vi "R45_2-FPGA.vi"() -> ()   [LabVIEW 2016]
uses:
  <vilib>/LabVIEW Targets/FPGA/cRIO/shared/nicrio_ModuleControls/nicrio_cRIO-9871_BaudRateEnum.ctl
  <vilib>/LabVIEW Targets/FPGA/cRIO/shared/nicrio_ModuleControls/nicrio_cRIO-9871_DataBitsEnum.ctl
  <vilib>/LabVIEW Targets/FPGA/cRIO/shared/nicrio_ModuleControls/nicrio_cRIO-9871_ParityEnum.ctl
  <vilib>/LabVIEW Targets/FPGA/cRIO/shared/nicrio_ModuleControls/nicrio_cRIO-9871_StopBitsEnum.ctl
  <vilib>/Platform/TimedLoop/XDataNode/timing_clust.ctl
  <vilib>/Platform/TimedLoop/XDataNode/nitl_modes.ctl
  <vilib>/Platform/TimedLoop/XDataNode/wakeup.ctl
  <vilib>/rvi/FXPMathLib/basic elements/FxpIntAccumulator/subVIs/nifxpmath_IntAccumulator_SimConfig.ctl
  <vilib>/rvi/Emulation/niFpgaGetClockAttributes.vi
  <vilib>/rvi/Emulation/niFpgaSctlEmulationGetInTimedLoop.vi
  <vilib>/rvi/Emulation/niFpgaEmulationReportErrorSimple.vi
  <vilib>/rvi/eio/common/nirviEmuTemplateMethod_errors.vi
  <vilib>/rvi/Emulation/niFpgaCriticalErrorInLSC.vi
  <vilib>/rvi/Analysis/common/codeGenErrors/XNode/niFpgaXNodeCodeGenErrorHandle.vi
  <vilib>/rvi/FXPMathLib/basic elements/FxpIntAccumulator/simVIs/DllFxpIntAccumulator_sub.vi
  <vilib>/rvi/eio/common/nirviEmuTemplatePropertySet_errors.vi
  <vilib>/eio/EIONode/EIONode.xnode
  <vilib>/rvi/Analysis/measure/dc-rms/XNode/niFpgaDC-RMS.xnode
  <vilib>/Platform/TimedLoop/XDataNode/XDataNode.xnode
  <vilib>/rvi/FXPMathLib/basic elements/FxpIntAccumulator/XNode/nifxpmath_IntAccumulator.xnode
  <vilib>/rvi/FXPMathLib/FxpMul/XNode/nifxpmath_Multiplier.xnode
  <vilib>/eio/EIOPropertyNode/EIOPropertyNode.xnode
  <vilib>/eio/EIOMethodNode/EIOMethodNode.xnode
  <vilib>/Platform/TimedLoop/XDataNode/XDNodeRunTimeDep.lvlib
  <vilib>/rvi/FXPMathLib/sim/FxpSim.dll
  <vilib>/rvi/eio/common/nirviEmuTemplatePropertyGet_errors.vi
  <vilib>/rvi/eio/common/nirviEmuTemplatePropertyGet_noerrors.vi
  <vilib>/rvi/eio/common/nirviEmuTemplatePropertySet_noerrors.vi
panel:
  out "Vac Cluster 2 interlock error":errorcluster
  out "ExB 2 PS error":errorcluster
  out "Position-Status Sensor error":errorcluster
  out "9485 error":errorcluster
  in  "RT error":bool
  out "R45 Vac Cluster 4 Ion Gauge 2":u8[](array[numeric])
  out "R45 Vac Cluster 4 Convectron 2":u8[](array[numeric])
  out "R45 Vac Cluster 4 Convectron 1":u8[](array[numeric])
  out "R45 Vac Cluster 4 Ion Gauge 1":u8[](array[numeric])
  out "R45 Vacuum Gauge 4 error":errorcluster
  out "R45 Vac Cluster 3 Ion Gauge 2":u8[](array[numeric])
  out "R45 Vac Cluster 3 Convectron 2":u8[](array[numeric])
  out "R45 Vac Cluster 3 Convectron 1":u8[](array[numeric])
  out "R45 Vac Cluster 3 Ion Gauge 1":u8[](array[numeric])
  out "R45 Vacuum Gauge 3 error":errorcluster
  out "R45 Vacuum Gauge 2 error":errorcluster
  out "GFM Hall Probe error":errorcluster
  out "GF ps error":errorcluster
  out "ExB 1 PS error":errorcluster
  out "9264 Error":errorcluster
  out "9205 error":errorcluster
  out "Vac cluster 2 Ion Guage Interlock":bool
  out "Vac cluster 2 Convectron Interlock":bool
  in  "turbo valve R45 ExB":bool
  in  "beamline valve R45 detector":bool
  in  "turbo valve r45 det turbo":bool
  in  "turbo valve r45 waist":bool
  out "Data":u8
  out "Timed Out":bool
  out "GFM read":u8[](array[numeric])
  in  "GFM ps set":u8[](array[numeric])=[0, 0, 0, 0, 0, 0, 0, 0, 0, 0]
  in  "ExB 2 Reset":bool
  in  "ExB 2 PS set":u8[](array[numeric])=[0, 0, 0, 0, 0, 0, 0, 0, 0, 0]
  out "R45 Vac Cluster 2 Ion Gauge 2":u8[](array[numeric])
  out "R45 Vac Cluster 2 Convectron 2":u8[](array[numeric])
  out "R45 Vac Cluster 2 Convectron 1":u8[](array[numeric])
  out "R45 Vac Cluster 2 Ion Gauge 1":u8[](array[numeric])
  in  "ExB 1 PS set":u8[](array[numeric])=[0, 0, 0, 0, 0, 0, 0, 0, 0, 0]
  out "DIO OUTPUT":bool[](array[boolean])
  in  "R45 detector FC insert":bool
  in  "R45 detector Aperture insert":bool
  out "Analog input":fxp<+/-,26,5>[](array[numeric]) format="%.23g"
  in  "Analog Output":fxp<+/-,26,5>[](array[numeric])=[0.0, 0.0, 0.0, 0.0, 0.0, 0.0, 0.0, 0.0] format="%.23g"
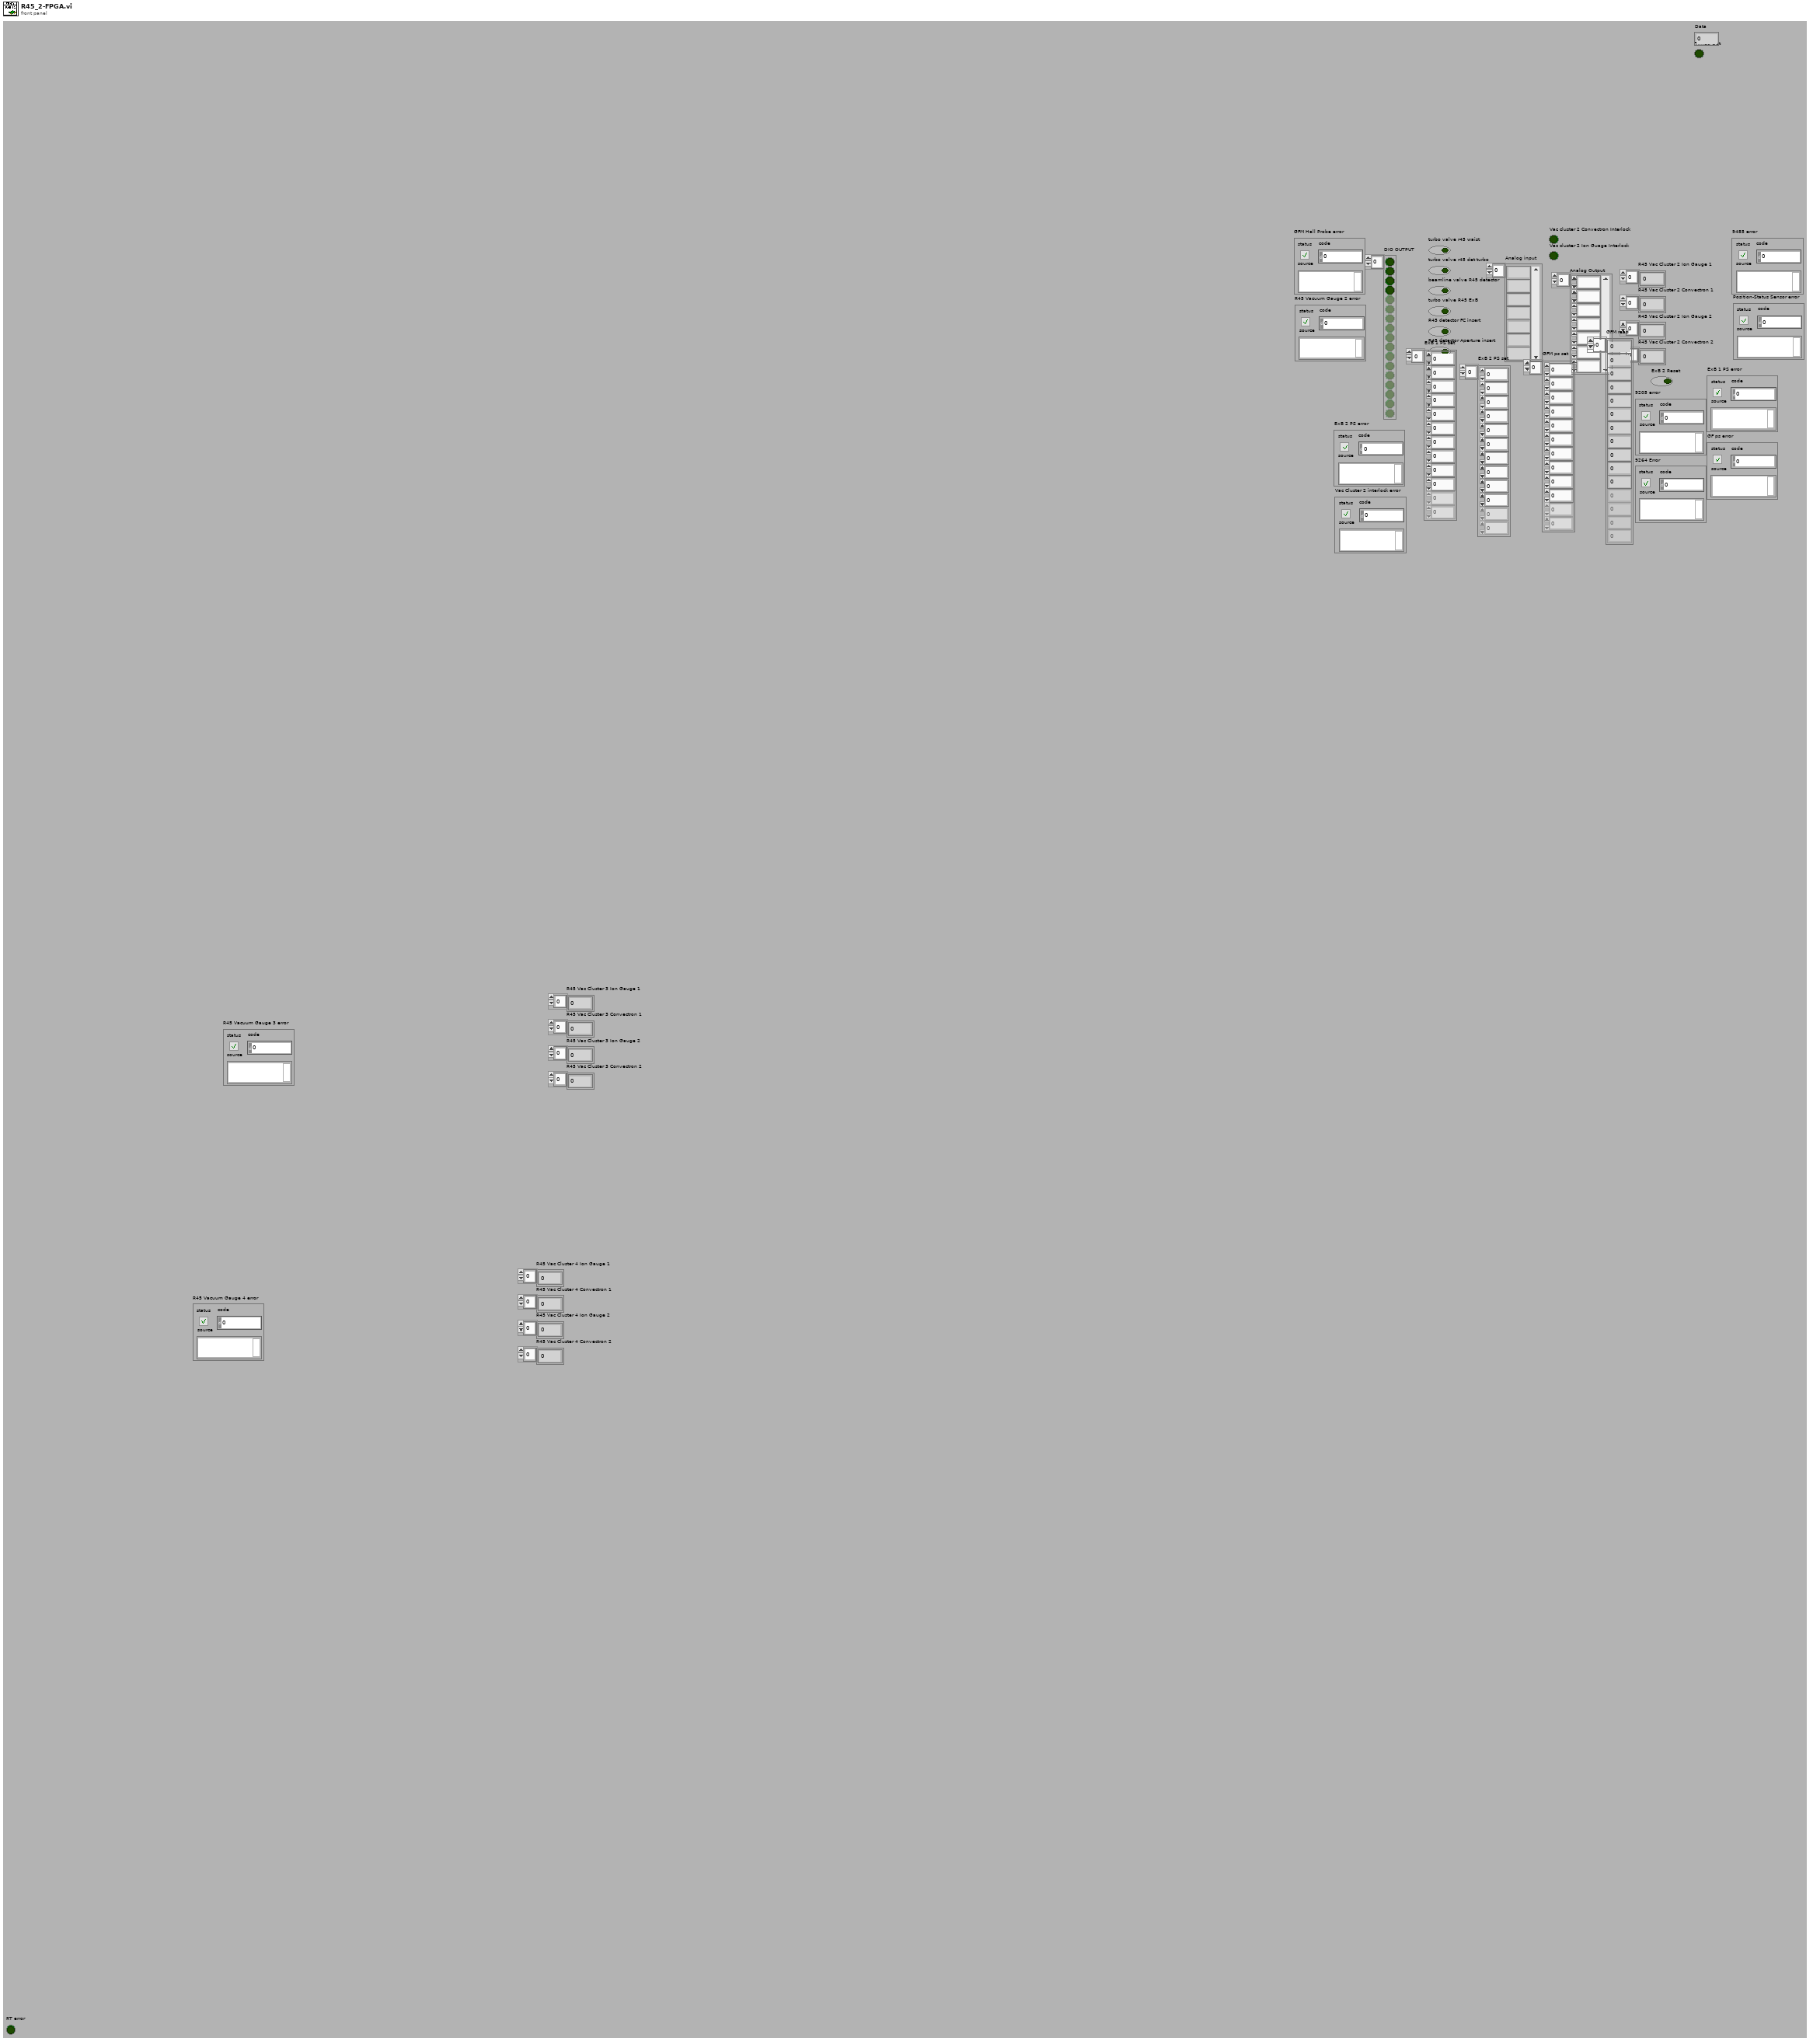
[diagram p1: front panel]
types:
  T1 = typedef "nicrio_cRIO-9871_StopBitsEnum.ctl" = enum8{"1", "1.5", "2"}
  T2 = typedef "nicrio_cRIO-9871_DataBitsEnum.ctl" = enum8{"5", "6", "7", "8"}
  T3 = typedef "nicrio_cRIO-9871_BaudRateEnum.ctl" = enum16{"75 bps", "110 bps", "134 bps", "150 bps", "300 bps", "600 bps", "1200 bps", "1800 bps", "2400 bps", "4800 bps", "7200 bps", "9600 bps", "14.4 kbps", "19.2 kbps", "28.8 kbps", "38.4 kbps", "57.6 kbps", "115.2 kbps", "230.4 kbps", "460.8 kbps", "921.6 kbps"}
  T4 = typedef "nicrio_cRIO-9871_ParityEnum.ctl" = enum8{"None", "Odd", "Even", "Mark", "Space"}
  T5 = typedef "XDNodeRunTimeDep.lvlib/timing_clust.ctl" = cluster{"Expected End [f-1]":u64, "Actual End [f-1]":u64, "Finished Late? [f-1]":bool, "Expected End [i-1]":u64, "Actual End [i-1]":u64, "Finished Late? [i-1]":bool, "Expected Start [i]":u64, "Actual Start [i]":u64, "Expected Start [f]":u64, "Actual Start [f]":u64, "Source Name":string, "Structure Name":string, "Period":i64, "Deadline":i64, "Offset":i64, "Start":i64, "Priority":i32, "Timeout":i32, "Mode":T6, "Wakeup Reason":T7, "Error":errorcluster, "Source Type":string, "Secondary Source Type":string, "Global End Time":u64, "Global Start Time":u64, "Frame Duration":u64, "Iteration Duration":u64, "Assigned CPU":i32, "I/O Scan Engine Mode":u32}
  T6 = typedef "XDNodeRunTimeDep.lvlib/nitl_modes.ctl" = enum32{"No Change", "Process missed periods, maintain original phase", "Discard missed periods, maintain original phase", "Process missed periods, ignore original phase", "Discard missed periods, ignore original phase"}
  T7 = typedef "XDNodeRunTimeDep.lvlib/wakeup.ctl" = enum32{"Normal", "Aborted", "Asynchronous wakeup", "Timing source error", "Timed loop error", "Timeout"}
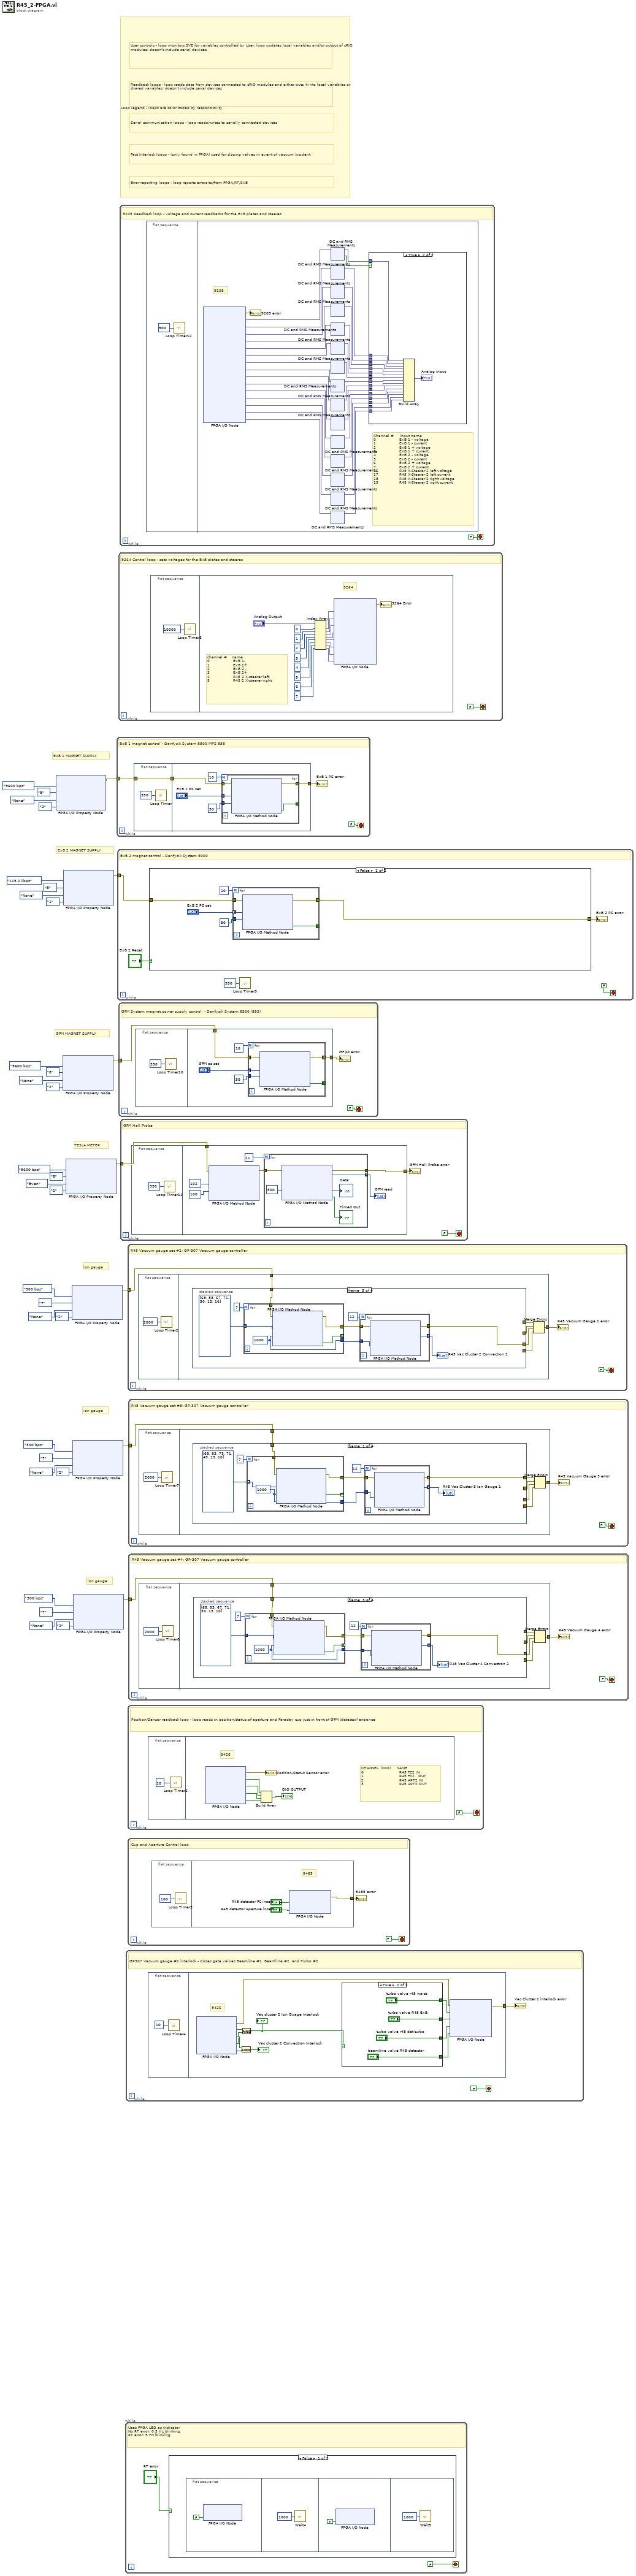
[diagram p0: block diagram]
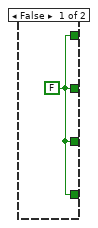
[diagram p2: hidden frame]
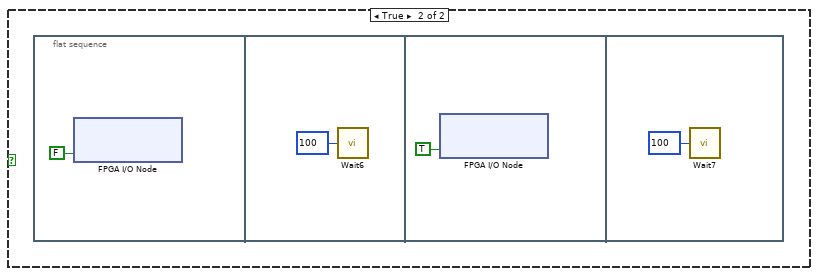
[diagram p3: hidden frame]
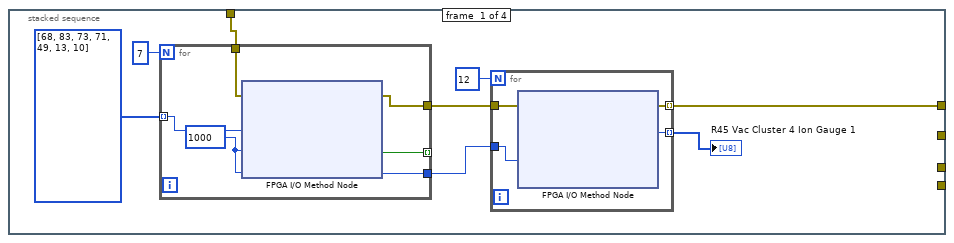
[diagram p4: hidden frame]
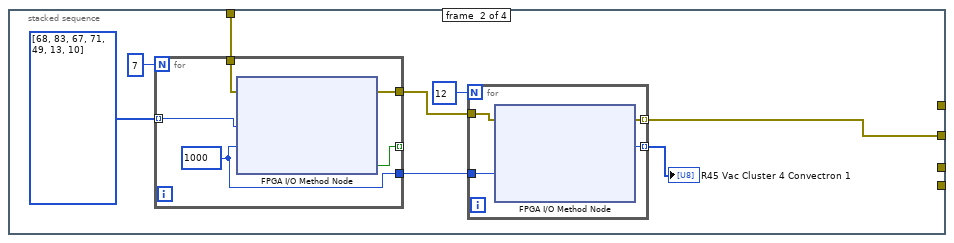
[diagram p5: hidden frame]
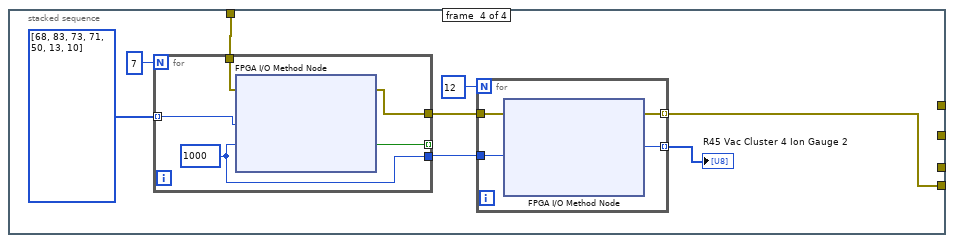
[diagram p6: hidden frame]
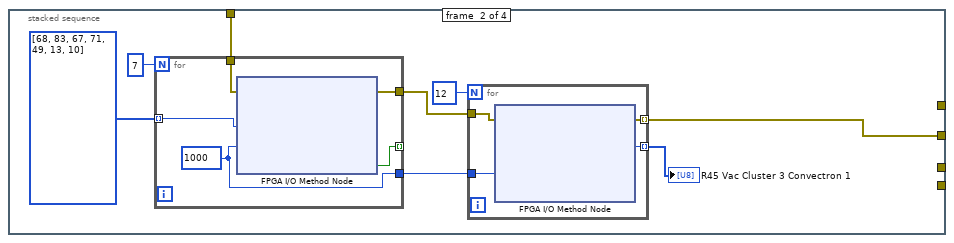
[diagram p7: hidden frame]
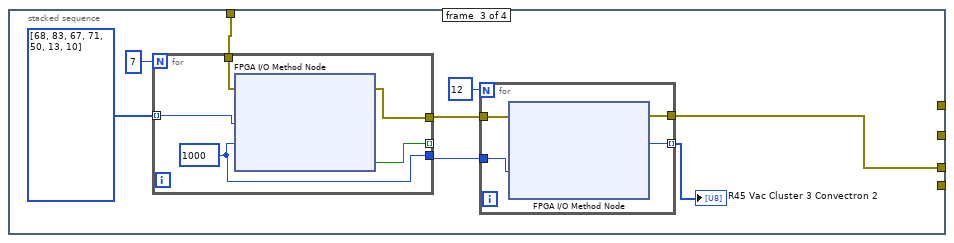
[diagram p8: hidden frame]
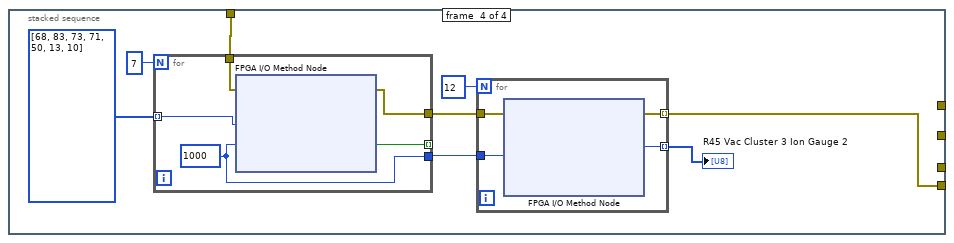
[diagram p9: hidden frame]
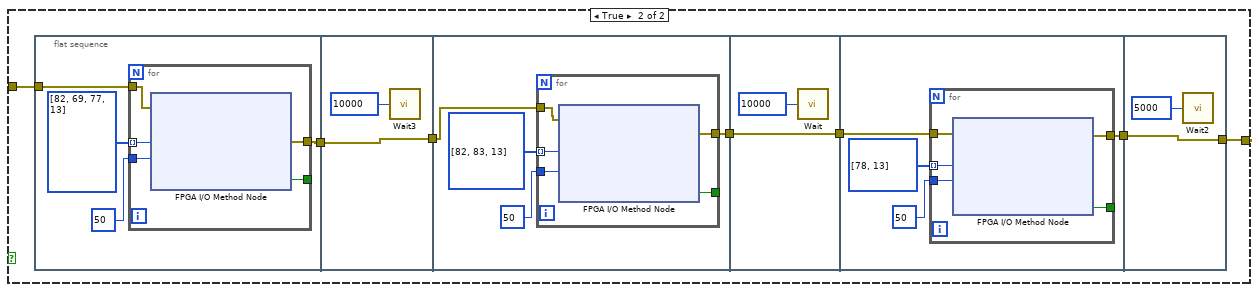
[diagram p11: hidden frame]
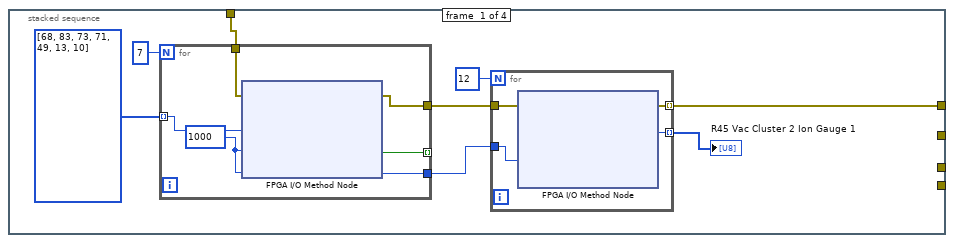
[diagram p12: hidden frame]
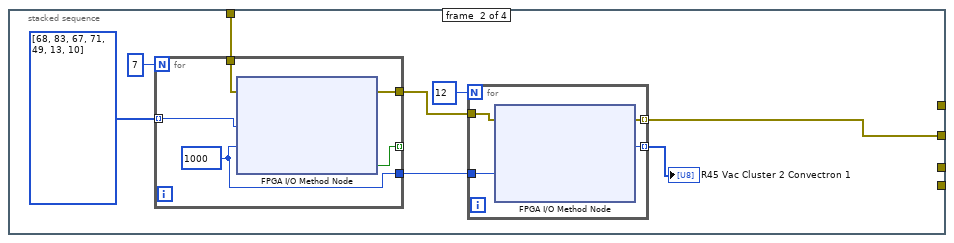
[diagram p13: hidden frame]
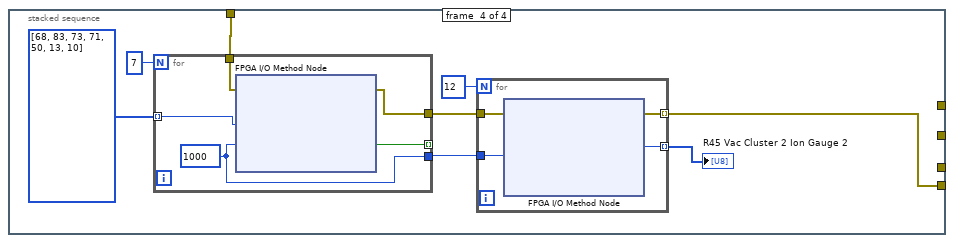
[diagram p14: hidden frame]
diagram:
  # "Fast Interlock loops - (only found in FPGA) used for closing valves in event of vacuum incident"
  # "Error reporting loops - loop reports errors to/from FPGA/RT/SVE"
  # "Serial communication loops - loop reads/writes to serially connected devices"
  # "Readback loops - loop reads data from devices connected to cRIO modules and either puts it into local variables or shared variables; doesn't include serial devices"
  # "User controls - loop monitors SVE for variables controlled by User; loop updates local variables and/or output of cRIO modules; doesn't include serial devices"
  # "Loop legend - loops are color coded by responsibility"
  # "TESLA METER"
  # "GFM MAGNET SUPPLY"
  # "ExB 2 MAGNET SUPPLY"
  # "ion gauge"
  # "ion gauge"
  # "ion gauge"
  # "ExB 1 MAGNET SUPPLY"
  n1 = xnode "FPGA I/O Property Node"("Baud Rate"=nicrio_cRIO-9871_BaudRateEnum."9600 bps", "Data Bits"=nicrio_cRIO-9871_DataBitsEnum."8", "Parity"=nicrio_cRIO-9871_ParityEnum."None", "Stop Bits"=nicrio_cRIO-9871_StopBitsEnum."2") -> ("error out"=w13:errorcluster)  [unwired: 2 in, 1 out]
  n2 = xnode "FPGA I/O Property Node"("Baud Rate"=nicrio_cRIO-9871_BaudRateEnum."9600 bps", "Data Bits"=nicrio_cRIO-9871_DataBitsEnum."8", "Parity"=nicrio_cRIO-9871_ParityEnum."None", "Stop Bits"=nicrio_cRIO-9871_StopBitsEnum."2") -> ("error out"=w8:errorcluster)  [unwired: 2 in, 1 out]
  n3 = xnode "FPGA I/O Property Node"("Baud Rate"=nicrio_cRIO-9871_BaudRateEnum."115.2 kbps", "Data Bits"=nicrio_cRIO-9871_DataBitsEnum."8", "Parity"=nicrio_cRIO-9871_ParityEnum."None", "Stop Bits"=nicrio_cRIO-9871_StopBitsEnum."1") -> ("error out"=w10:errorcluster)  [unwired: 2 in, 1 out]
  n4 = xnode "FPGA I/O Property Node"("Baud Rate"=nicrio_cRIO-9871_BaudRateEnum."9600 bps", "Data Bits"=nicrio_cRIO-9871_DataBitsEnum."8", "Parity"=nicrio_cRIO-9871_ParityEnum."Even", "Stop Bits"=nicrio_cRIO-9871_StopBitsEnum."1") -> ("error out"=w4:errorcluster)  [unwired: 2 in, 1 out]
  n5 = xnode "FPGA I/O Property Node"("Baud Rate"=nicrio_cRIO-9871_BaudRateEnum."300 bps", "Data Bits"=nicrio_cRIO-9871_DataBitsEnum."7", "Parity"=nicrio_cRIO-9871_ParityEnum."None", "Stop Bits"=nicrio_cRIO-9871_StopBitsEnum."2") -> ("error out"=w3:errorcluster)  [unwired: 2 in, 1 out]
  n6 = xnode "FPGA I/O Property Node"("Baud Rate"=nicrio_cRIO-9871_BaudRateEnum."300 bps", "Data Bits"=nicrio_cRIO-9871_DataBitsEnum."7", "Parity"=nicrio_cRIO-9871_ParityEnum."None", "Stop Bits"=nicrio_cRIO-9871_StopBitsEnum."2") -> ("error out"=w2:errorcluster)  [unwired: 2 in, 1 out]
  n7 = xnode "FPGA I/O Property Node"("Baud Rate"=nicrio_cRIO-9871_BaudRateEnum."300 bps", "Data Bits"=nicrio_cRIO-9871_DataBitsEnum."7", "Parity"=nicrio_cRIO-9871_ParityEnum."None", "Stop Bits"=nicrio_cRIO-9871_StopBitsEnum."2") -> ("error out"=w1:errorcluster)  [unwired: 2 in, 1 out]
  n8 = while {
    tunnel: w13 -> [w36]
    stop <- FALSE stop-if-true
    # "ExB 1 magnet control - Danfysik System 8500 MPS 858"
    n9 = flat-sequence {
      tunnel: [w40] -> w37
      tunnel: w36 -> [w40]
      tunnel: [w43] -> w38
      tunnel: w37 -> [w42]
      frame #0 {
        n10 = call "Loop Timer"("Count(mSec)"=u32 350) -> ()  [unwired: 1 out]
      }
      frame #1 {
        n11 = for {
          N: 10 -> [_]
          tunnel: 50 ("Timeout (ms)") -> [w51]
          tunnel: "ExB 1 PS set" -> [w50] mode=indexing
          tunnel: [w47] -> _
          tunnel: w42 -> [w49]
          tunnel: [w48] -> w43
          n12 = xnode "FPGA I/O Method Node"("error in"=w49, "Data"=w50, "Timeout (ms)"=w51) -> ("error out"=w48:errorcluster, "Timed Out"=w47:bool)  [unwired: 1 in, 1 out]
        }
      }
    }
    "ExB 1 PS error" <- w38
  }
  n13 = while {
    tunnel: w10 -> [w53]
    stop <- FALSE stop-if-true
    # "ExB 2 magnet control - Danfysik System 9000"
    n14 = case shown="False" "ExB 2 Reset" {
      tunnel: w53 -> [w58 w73]
      tunnel: [w57 w67] -> w52
      frame False {
        n15 = for {
          N: 10 -> [_]
          tunnel: 50 ("Timeout (ms)") -> [w66]
          tunnel: "ExB 2 PS set" -> [w65] mode=indexing
          tunnel: [w64] -> _
          tunnel: w58 -> [w63]
          tunnel: [w62] -> w57
          n16 = xnode "FPGA I/O Method Node"("error in"=w63, "Data"=w65, "Timeout (ms)"=w66) -> ("error out"=w62:errorcluster, "Timed Out"=w64:bool)  [unwired: 1 in, 1 out]
        }
      }
      frame True {
        n17 = flat-sequence {
          tunnel: w73 -> [w75]
          tunnel: [w74] -> w71
          tunnel: [w83] -> w72
          tunnel: w71 -> [w83]
          tunnel: w72 -> [w86]
          tunnel: [w85] -> w69
          tunnel: [w94] -> w70
          tunnel: w69 -> [w94]
          tunnel: w70 -> [w97]
          tunnel: [w96] -> w68
          tunnel: w68 -> [w105]
          tunnel: [w105] -> w67
          frame #0 {
            n18 = for {
              tunnel: 50 ("Timeout (ms)") -> [w82]
              tunnel: u8[] [82, 69, 77, 13] ("unsigned byte array") -> [w81] mode=indexing
              tunnel: [w80] -> _
              tunnel: w75 -> [w79]
              tunnel: [w78] -> w74
              n19 = xnode "FPGA I/O Method Node"("error in"=w79, "Data"=w81, "Timeout (ms)"=w82) -> ("error out"=w78:errorcluster, "Timed Out"=w80:bool)  [unwired: 1 in, 1 out]
            }
          }
          frame #1 {
            n20 = call "Wait3"("Count(mSec)"=u32 10000) -> ()  [unwired: 1 out]
          }
          frame #2 {
            n21 = for {
              tunnel: 50 ("Timeout (ms)") -> [w93]
              tunnel: u8[] [82, 83, 13] ("unsigned byte array") -> [w92] mode=indexing
              tunnel: [w91] -> _
              tunnel: w86 -> [w89]
              tunnel: [w90] -> w85
              n22 = xnode "FPGA I/O Method Node"("error in"=w89, "Data"=w92, "Timeout (ms)"=w93) -> ("error out"=w90:errorcluster, "Timed Out"=w91:bool)  [unwired: 1 in, 1 out]
            }
          }
          frame #3 {
            n23 = call "Wait"("Count(mSec)"=u32 10000) -> ()  [unwired: 1 out]
          }
          frame #4 {
            n24 = for {
              tunnel: 50 ("Timeout (ms)") -> [w104]
              tunnel: u8[] [78, 13] ("unsigned byte array") -> [w103] mode=indexing
              tunnel: [w102] -> _
              tunnel: w97 -> [w101]
              tunnel: [w100] -> w96
              n25 = xnode "FPGA I/O Method Node"("error in"=w101, "Data"=w103, "Timeout (ms)"=w104) -> ("error out"=w100:errorcluster, "Timed Out"=w102:bool)  [unwired: 1 in, 1 out]
            }
          }
          frame #5 {
            n26 = call "Wait2"("Count(mSec)"=u32 5000) -> ()  [unwired: 1 out]
          }
        }
      }
    }
    "ExB 2 PS error" <- w52
    n27 = call "Loop Timer9"("Count(mSec)"=u32 350) -> ()  [unwired: 1 out]
  }
  n28 = while {
    stop <- FALSE stop-if-true
    # "9264 Control loop - sets voltages for the ExB plates and steeres"
    n29 = flat-sequence {
      frame #0 {
        n30 = call "Loop Timer3"("Count(Ticks)"=u32 10000) -> ()  [unwired: 1 out]
      }
      frame #1 {
        # "9264"
        # "channel #    name\n0                   ExB 1-\n1                   ExB 1+\n2                   ExB 2 -\n3                   ExB 2+\n4                   R45 2 X-steerer left\n5                   R45 2 X-steerer right"
        n31 = Index Array(array="Analog Output", index #1=0 ("index"), index #2=1 ("index"), index #3=2 ("index"), index #4=3 ("index"), index #5=4 ("index"), index #6=5 ("index"), index #7=6 ("index"), index #8=7 ("index")) -> (element #1=w121:fxp<+/-,26,5>, element #2=w120:fxp<+/-,26,5>, element #3=w119:fxp<+/-,26,5>, element #4=w118:fxp<+/-,26,5>, element #5=w113:fxp<+/-,26,5>, element #6=w112:fxp<+/-,26,5>, element #7=w111:fxp<+/-,26,5>, element #8=w110:fxp<+/-,26,5>)
        n32 = xnode "FPGA I/O Node"("Mod2/AO0"=w121, "Mod2/AO1"=w120, "Mod2/AO2"=w119, "Mod2/AO3"=w118, "Mod2/AO4"=w113, "Mod2/AO5"=w112, "Mod2/AO6"=w111, "Mod2/AO7"=w110) -> ("error out"=→"9264 Error":errorcluster)  [unwired: 9 in, 8 out]
      }
    }
  }
  n33 = while {
    tunnel: w8 -> [w128]
    stop <- FALSE stop-if-true
    # "GFM System magnet power supply control  - Danfysik System 8500 (853)"
    n34 = flat-sequence {
      tunnel: w128 -> [w132]
      tunnel: [w131] -> w127
      frame #0 {
        n35 = call "Loop Timer10"("Count(mSec)"=u32 350) -> ()  [unwired: 1 out]
      }
      frame #1 {
        n36 = for {
          N: 10 -> [_]
          tunnel: 50 ("Timeout (ms)") -> [w137]
          tunnel: "GFM ps set" -> [w138] mode=indexing
          tunnel: w132 -> [w140]
          tunnel: [w139] -> w131
          tunnel: [w136] -> _
          n37 = xnode "FPGA I/O Method Node"("error in"=w140, "Data"=w138, "Timeout (ms)"=w137) -> ("error out"=w139:errorcluster, "Timed Out"=w136:bool)  [unwired: 1 in, 1 out]
        }
      }
    }
    "GF ps error" <- w127
  }
  n38 = while {
    stop <- FALSE stop-if-true
    # "9205 Readback loop - voltage and current readbacks for the ExB plates and steeres"
    n39 = flat-sequence {
      frame #0 {
        n40 = call "Loop Timer12"("Count(Ticks)"=u32 500) -> ()  [unwired: 1 out]
      }
      frame #1 {
        # "Channel #     input name\n0                   ExB 1 - voltage\n1                   ExB 1 - current\n2                   ExB 1 + voltage\n3                   ExB 1 + current\n4                   ExB 2 - voltage\n5                   ExB 2 - current\n6                   ExB 2 + voltage\n7                   ExB 2 + current                   \n16                 R45 X-Steerer 2 left voltage\n17                 R45 X-Steerer 2 left current\n18                 R45 X-Steerer 2 right voltage\n19                 R45 X-Steerer 2 right current"
        # "9205"
        n41 = xnode "FPGA I/O Node"() -> ("error out"=→"9205 error":errorcluster, "Mod1/AI0"=w173:fxp<+/-,26,5>, "Mod1/AI1"=w171:fxp<+/-,26,5>, "Mod1/AI2"=w169:fxp<+/-,26,5>, "Mod1/AI3"=w167:fxp<+/-,26,5>, "Mod1/AI4"=w165:fxp<+/-,26,5>, "Mod1/AI5"=w163:fxp<+/-,26,5>, "Mod1/AI6"=w161:fxp<+/-,26,5>, "Mod1/AI7"=w159:fxp<+/-,26,5>, "Mod1/AI16"=w157:fxp<+/-,26,5>, "Mod1/AI17"=w155:fxp<+/-,26,5>, "Mod1/AI18"=w153:fxp<+/-,26,5>, "Mod1/AI19"=w151:fxp<+/-,26,5>, "Mod1/AI20"=w149:fxp<+/-,26,5>, "Mod1/AI21"=w147:fxp<+/-,26,5>, "Mod1/AI22"=w145:fxp<+/-,26,5>)  [unwired: 16 in, 15 out]
        n42 = xnode "DC and RMS Measurements"("input data"=w173) -> ("DC"=w172:fxp<+/-,26,5>, "output valid"=w174:bool)  [unwired: 1 in]
        n43 = xnode "DC and RMS Measurements"("input data"=w171) -> ("DC"=w170:fxp<+/-,26,5>)  [unwired: 1 in, 1 out]
        n44 = xnode "DC and RMS Measurements"("input data"=w169) -> ("DC"=w168:fxp<+/-,26,5>)  [unwired: 1 in, 1 out]
        n45 = xnode "DC and RMS Measurements"("input data"=w167) -> ("DC"=w166:fxp<+/-,26,5>)  [unwired: 1 in, 1 out]
        n46 = xnode "DC and RMS Measurements"("input data"=w165) -> ("DC"=w164:fxp<+/-,26,5>)  [unwired: 1 in, 1 out]
        n47 = xnode "DC and RMS Measurements"("input data"=w163) -> ("DC"=w162:fxp<+/-,26,5>)  [unwired: 1 in, 1 out]
        n48 = xnode "DC and RMS Measurements"("input data"=w161) -> ("DC"=w160:fxp<+/-,26,5>)  [unwired: 1 in, 1 out]
        n49 = xnode "DC and RMS Measurements"("input data"=w159) -> ("DC"=w158:fxp<+/-,26,5>)  [unwired: 1 in, 1 out]
        n50 = xnode "DC and RMS Measurements"("input data"=w157) -> ("DC"=w156:fxp<+/-,26,5>)  [unwired: 1 in, 1 out]
        n51 = xnode "DC and RMS Measurements"("input data"=w155) -> ("DC"=w154:fxp<+/-,26,5>)  [unwired: 1 in, 1 out]
        n52 = xnode "DC and RMS Measurements"("input data"=w153) -> ("DC"=w152:fxp<+/-,26,5>)  [unwired: 1 in, 1 out]
        n53 = xnode "DC and RMS Measurements"("input data"=w151) -> ("DC"=w150:fxp<+/-,26,5>)  [unwired: 1 in, 1 out]
        n54 = xnode "DC and RMS Measurements"("input data"=w149) -> ("DC"=w148:fxp<+/-,26,5>)  [unwired: 1 in, 1 out]
        n55 = xnode "DC and RMS Measurements"("input data"=w147) -> ("DC"=w146:fxp<+/-,26,5>)  [unwired: 1 in, 1 out]
        n56 = xnode "DC and RMS Measurements"("input data"=w145) -> ("DC"=w144:fxp<+/-,26,5>)  [unwired: 1 in, 1 out]
        n57 = case shown="True" w174 {
          tunnel: w172 -> [_ w350]
          tunnel: w170 -> [_ w349]
          tunnel: w168 -> [_ w348]
          tunnel: w166 -> [_ w347]
          tunnel: w164 -> [_ w346]
          tunnel: w162 -> [_ w345]
          tunnel: w160 -> [_ w344]
          tunnel: w158 -> [_ w343]
          tunnel: w156 -> [_ w342]
          tunnel: w154 -> [_ w341]
          tunnel: w152 -> [_ w340]
          tunnel: w150 -> [_ w339]
          tunnel: w148 -> [_ w338]
          tunnel: w146 -> [_ w337]
          tunnel: w144 -> [_ w336]
          frame False {
          }
          frame True {
            n58 = Build Array(w350, w349, w348, w347, w346, w345, w344, w343, w342, w341, w340, w339, w338, w337, w336) -> (→"Analog input":fxp<+/-,26,5>[])
          }
        }
      }
    }
  }
  n59 = while {
    tunnel: w4 -> [w1392]
    stop <- FALSE stop-if-true
    # "GFM Hall Probe"
    n60 = flat-sequence {
      tunnel: w1392 -> [w1398]
      tunnel: [w1397] -> w1391
      frame #0 {
        n61 = call "Loop Timer11"("Count(mSec)"=u32 350) -> ()  [unwired: 1 out]
      }
      frame #1 {
        n62 = xnode "FPGA I/O Method Node"("error in"=w1398, "Data"=u8 102, "Timeout (ms)"=100) -> ("error out"=w1399:errorcluster)  [unwired: 1 in, 2 out]
        n63 = for {
          N: 11 ("Numeric 3") -> [_]
          tunnel: [w1405] -> w1395 mode=indexing
          tunnel: w1399 -> [w1404]
          tunnel: [w1403] -> w1397
          n64 = xnode "FPGA I/O Method Node"("error in"=w1404, "Timeout (ms)"=500) -> ("error out"=w1403:errorcluster, "Data"=w1405:u8, "Timed Out"=→"Timed Out":bool)  [unwired: 1 in, 1 out]
          "Data" <- w1405
        }
        "GFM read" <- w1395
      }
    }
    "GFM Hall Probe error" <- w1391
  }
  n65 = while {
    stop <- FALSE stop-if-true
    # "Uses FPGA LED as indicator\nNo RT error: 0.5 Hz blinking\nRT error: 5 Hz blinking"
    n66 = case shown="False" "RT error" {
      frame False {
        n67 = flat-sequence {
          frame #0 {
            n68 = xnode "FPGA I/O Node"("FPGA LED"=FALSE) -> ()  [unwired: 1 in, 1 out]
          }
          frame #1 {
            n69 = call "Wait4"("Count(mSec)"=u16 1000) -> ()  [unwired: 1 out]
          }
          frame #2 {
            n70 = xnode "FPGA I/O Node"("FPGA LED"=TRUE) -> ()  [unwired: 1 in, 1 out]
          }
          frame #3 {
            n71 = call "Wait5"("Count(mSec)"=u16 1000) -> ()  [unwired: 1 out]
          }
        }
      }
      frame True {
        n72 = flat-sequence {
          frame #0 {
            n73 = xnode "FPGA I/O Node"("FPGA LED"=FALSE) -> ()  [unwired: 1 in, 1 out]
          }
          frame #1 {
            n74 = call "Wait6"("Count(mSec)"=u16 100) -> ()  [unwired: 1 out]
          }
          frame #2 {
            n75 = xnode "FPGA I/O Node"("FPGA LED"=TRUE) -> ()  [unwired: 1 in, 1 out]
          }
          frame #3 {
            n76 = call "Wait7"("Count(mSec)"=u16 100) -> ()  [unwired: 1 out]
          }
        }
      }
    }
  }
  n77 = while {
    stop <- FALSE stop-if-true
    # "GP307 Vacuum gauge #2 interlock - closes gate valves Beamline #1, Beamline #2, and Turbo #2"
    n78 = flat-sequence {
      tunnel: [w1420] -> w1417
      frame #0 {
        n79 = call "Loop Timer4"("Count(uSec)"=u32 10 ("Count(Ticks)")) -> ()  [unwired: 1 out]
      }
      frame #1 {
        # "9426"
        n80 = xnode "FPGA I/O Node"() -> ("error out"=w1421:errorcluster, "Mod7/DI5"=w1424:bool, "Mod7/DI6"=w1431:bool, "Mod7/DI7"=w1423:bool, "Mod7/DI8"=w1430:bool)  [unwired: 5 in, 4 out]
        n81 = And(x=w1431, y=w1430) -> (x .and. y?=→"Vac cluster 2 Convectron Interlock":bool)
        n82 = And(x=w1424, y=w1423) -> (x .and. y?=w1422:bool)
        "Vac cluster 2 Ion Guage Interlock" <- w1422
        n83 = case shown="True" w1422 {
          tunnel: [w1432 "turbo valve r45 waist"] -> w1429
          tunnel: [w1432 "turbo valve R45 ExB"] -> w1428
          tunnel: [w1432 "turbo valve r45 det turbo"] -> w1427
          tunnel: [w1432 "beamline valve R45 detector"] -> w1426
          frame False {
            w1432 = FALSE ("turbo valve r45 waist")
          }
          frame True {
          }
        }
        n84 = xnode "FPGA I/O Node"("error in"=w1421, "Mod8/CH3"=w1429, "Mod8/CH4"=w1428, "Mod8/CH5"=w1427, "Mod8/CH6"=w1426) -> ("error out"=w1420:errorcluster)  [unwired: 4 in, 4 out]
      }
    }
    "Vac Cluster 2 interlock error" <- w1417
  }
  n85 = while {
    tunnel: w3 -> [w1438]
    stop <- FALSE stop-if-true
    # "R45 Vacuum gauge set #2: GP-307 Vacuum gauge controller"
    n86 = flat-sequence {
      tunnel: w1438 -> [w1446]
      tunnel: [w1441] -> w1437
      frame #0 {
        n87 = call "Loop Timer2"("Count(mSec)"=u32 2000 ("Count(Ticks)")) -> ()  [unwired: 1 out]
      }
      frame #1 {
        n88 = stacked-sequence {
          tunnel: [_ _ w1483 _] -> w1443
          tunnel: [_ _ _ w1499] -> w1442
          tunnel: w1446 -> [w1449 w1466 w1481 w1498]
          tunnel: [w1447 _ _ _] -> w1445
          tunnel: [_ w1465 _ _] -> w1444
          frame #0 {
            n89 = for {
              N: 7 -> [_]
              tunnel: [w1463] -> w1450
              tunnel: [w1462] -> _ mode=indexing
              tunnel: u8[] [68, 83, 73, 71, 49, 13, 10] ("unsigned byte array") -> [w1461] mode=indexing
              tunnel: w1449 -> [w1460]
              tunnel: [w1459] -> w1448
              w1463 = 1000 ("Timeout (ms)")
              n90 = xnode "FPGA I/O Method Node"("error in"=w1460, "Data"=w1461, "Timeout (ms)"=w1463) -> ("error out"=w1459:errorcluster, "Timed Out"=w1462:bool)  [unwired: 1 in, 1 out]
            }
            n91 = for {
              N: 12 -> [_]
              tunnel: w1450 -> [w1458]
              tunnel: [w1457] -> w1451 mode=indexing
              tunnel: w1448 -> [w1456]
              tunnel: [w1455] -> w1447 mode=indexing
              n92 = xnode "FPGA I/O Method Node"("error in"=w1456, "Timeout (ms)"=w1458) -> ("error out"=w1455:errorcluster, "Data"=w1457:u8)  [unwired: 1 in, 2 out]
            }
            "R45 Vac Cluster 2 Ion Gauge 1" <- w1451
          }
          frame #1 {
            n93 = for {
              N: 7 -> [_]
              tunnel: [w1479] -> w1471
              tunnel: [w1478] -> _ mode=indexing
              tunnel: u8[] [68, 83, 67, 71, 49, 13, 10] ("unsigned byte array") -> [w1480] mode=indexing
              tunnel: w1466 -> [w1477]
              tunnel: [w1476] -> w1464
              w1479 = 1000 ("Timeout (ms)")
              n94 = xnode "FPGA I/O Method Node"("error in"=w1477, "Data"=w1480, "Timeout (ms)"=w1479) -> ("error out"=w1476:errorcluster, "Timed Out"=w1478:bool)  [unwired: 1 in, 1 out]
            }
            n95 = for {
              N: 12 -> [_]
              tunnel: w1471 -> [w1475]
              tunnel: [w1474] -> w1467 mode=indexing
              tunnel: w1464 -> [w1473]
              tunnel: [w1472] -> w1465 mode=indexing
              n96 = xnode "FPGA I/O Method Node"("error in"=w1473, "Timeout (ms)"=w1475) -> ("error out"=w1472:errorcluster, "Data"=w1474:u8)  [unwired: 1 in, 2 out]
            }
            "R45 Vac Cluster 2 Convectron 1" <- w1467
          }
          frame #2 {
            n97 = for {
              N: 7 -> [_]
              tunnel: [w1495] -> w1488
              tunnel: [w1496] -> _ mode=indexing
              tunnel: u8[] [68, 83, 67, 71, 50, 13, 10] ("unsigned byte array") -> [w1497] mode=indexing
              tunnel: [w1494] -> w1484
              tunnel: w1481 -> [w1493]
              w1495 = 1000 ("Timeout (ms)")
              n98 = xnode "FPGA I/O Method Node"("error in"=w1493, "Data"=w1497, "Timeout (ms)"=w1495) -> ("error out"=w1494:errorcluster, "Timed Out"=w1496:bool)  [unwired: 1 in, 1 out]
            }
            n99 = for {
              N: 12 -> [_]
              tunnel: w1488 -> [w1492]
              tunnel: [w1491] -> w1482 mode=indexing
              tunnel: w1484 -> [w1490]
              tunnel: [w1489] -> w1483
              n100 = xnode "FPGA I/O Method Node"("error in"=w1490, "Timeout (ms)"=w1492) -> ("error out"=w1489:errorcluster, "Data"=w1491:u8)  [unwired: 1 in, 2 out]
            }
            "R45 Vac Cluster 2 Convectron 2" <- w1482
          }
          frame #3 {
            n101 = for {
              N: 7 -> [_]
              tunnel: [w1512] -> w1505
              tunnel: [w1514] -> _ mode=indexing
              tunnel: u8[] [68, 83, 73, 71, 50, 13, 10] ("unsigned byte array") -> [w1513] mode=indexing
              tunnel: [w1511] -> w1500
              tunnel: w1498 -> [w1510]
              w1512 = 1000 ("Timeout (ms)")
              n102 = xnode "FPGA I/O Method Node"("error in"=w1510, "Data"=w1513, "Timeout (ms)"=w1512) -> ("error out"=w1511:errorcluster, "Timed Out"=w1514:bool)  [unwired: 1 in, 1 out]
            }
            n103 = for {
              N: 12 -> [_]
              tunnel: w1505 -> [w1509]
              tunnel: [w1508] -> w1501 mode=indexing
              tunnel: w1500 -> [w1507]
              tunnel: [w1506] -> w1499 mode=indexing
              n104 = xnode "FPGA I/O Method Node"("error in"=w1507, "Timeout (ms)"=w1509) -> ("error out"=w1506:errorcluster, "Data"=w1508:u8)  [unwired: 1 in, 2 out]
            }
            "R45 Vac Cluster 2 Ion Gauge 2" <- w1501
          }
        }
        n105 = Merge Errors(w1445, w1444, w1443, w1442) -> (w1441:errorcluster)
      }
    }
    "R45 Vacuum Gauge 2 error" <- w1437
  }
  n106 = while {
    stop <- FALSE stop-if-true
    # "Position/Sensor readback loop - loop reads in position/status of aperture and Faraday cup just in front of GFM (detector) entrance"
    n107 = flat-sequence {
      frame #0 {
        n108 = call "Loop Timer6"("Count(uSec)"=u32 10 ("Count(Ticks)")) -> ()  [unwired: 1 out]
      }
      frame #1 {
        # "CHANNEL  (DIO)     NAME\n0                             R45 FC2 IN\n1                             R45 FC2   OUT\n2                             R45 APT2 IN\n3                             R45 APT2 OUT"
        # "9426"
        n109 = xnode "FPGA I/O Node"() -> ("error out"=→"Position-Status Sensor error":errorcluster, "Mod7/DI0"=w1518:bool, "Mod7/DI1"=w1519:bool, "Mod7/DI2"=w1520:bool, "Mod7/DI3"=w1521:bool)  [unwired: 5 in, 4 out]
        n110 = Build Array(w1518, w1519, w1520, w1521) -> (→"DIO OUTPUT":bool[])
      }
    }
  }
  n111 = while {
    stop <- FALSE stop-if-true
    # "Cup and Aperture Control loop"
    n112 = flat-sequence {
      tunnel: [w1526] -> w1523
      frame #0 {
        n113 = call "Loop Timer5"("Count(uSec)"=u32 100 ("Count(Ticks)")) -> ()  [unwired: 1 out]
      }
      frame #1 {
        # "9485"
        n114 = xnode "FPGA I/O Node"("Mod8/CH0"="R45 detector FC insert", "Mod8/CH2"="R45 detector Aperture insert") -> ("error out"=w1526:errorcluster)  [unwired: 3 in, 2 out]
      }
    }
    "9485 error" <- w1523
  }
  n115 = while {
    tunnel: w2 -> [w1530]
    stop <- FALSE stop-if-true
    # "R45 Vacuum gauge set #3: GP-307 Vacuum gauge controller"
    n116 = flat-sequence {
      tunnel: w1530 -> [w1538]
      tunnel: [w1533] -> w1529
      frame #0 {
        n117 = call "Loop Timer7"("Count(mSec)"=u32 2000 ("Count(Ticks)")) -> ()  [unwired: 1 out]
      }
      frame #1 {
        n118 = stacked-sequence {
          tunnel: [_ _ w1575 _] -> w1535
          tunnel: [_ _ _ w1591] -> w1534
          tunnel: w1538 -> [w1541 w1558 w1573 w1590]
          tunnel: [w1539 _ _ _] -> w1537
          tunnel: [_ w1557 _ _] -> w1536
          frame #0 {
            n119 = for {
              N: 7 -> [_]
              tunnel: [w1555] -> w1542
              tunnel: [w1554] -> _ mode=indexing
              tunnel: u8[] [68, 83, 73, 71, 49, 13, 10] ("unsigned byte array") -> [w1553] mode=indexing
              tunnel: w1541 -> [w1552]
              tunnel: [w1551] -> w1540
              w1555 = 1000 ("Timeout (ms)")
              n120 = xnode "FPGA I/O Method Node"("error in"=w1552, "Data"=w1553, "Timeout (ms)"=w1555) -> ("error out"=w1551:errorcluster, "Timed Out"=w1554:bool)  [unwired: 1 in, 1 out]
            }
            n121 = for {
              N: 12 -> [_]
              tunnel: w1542 -> [w1550]
              tunnel: [w1549] -> w1543 mode=indexing
              tunnel: w1540 -> [w1548]
              tunnel: [w1547] -> w1539 mode=indexing
              n122 = xnode "FPGA I/O Method Node"("error in"=w1548, "Timeout (ms)"=w1550) -> ("error out"=w1547:errorcluster, "Data"=w1549:u8)  [unwired: 1 in, 2 out]
            }
            "R45 Vac Cluster 3 Ion Gauge 1" <- w1543
          }
          frame #1 {
            n123 = for {
              N: 7 -> [_]
              tunnel: [w1571] -> w1563
              tunnel: [w1570] -> _ mode=indexing
              tunnel: u8[] [68, 83, 67, 71, 49, 13, 10] ("unsigned byte array") -> [w1572] mode=indexing
              tunnel: w1558 -> [w1569]
              tunnel: [w1568] -> w1556
              w1571 = 1000 ("Timeout (ms)")
              n124 = xnode "FPGA I/O Method Node"("error in"=w1569, "Data"=w1572, "Timeout (ms)"=w1571) -> ("error out"=w1568:errorcluster, "Timed Out"=w1570:bool)  [unwired: 1 in, 1 out]
            }
            n125 = for {
              N: 12 -> [_]
              tunnel: w1563 -> [w1567]
              tunnel: [w1566] -> w1559 mode=indexing
              tunnel: w1556 -> [w1565]
              tunnel: [w1564] -> w1557 mode=indexing
              n126 = xnode "FPGA I/O Method Node"("error in"=w1565, "Timeout (ms)"=w1567) -> ("error out"=w1564:errorcluster, "Data"=w1566:u8)  [unwired: 1 in, 2 out]
            }
            "R45 Vac Cluster 3 Convectron 1" <- w1559
          }
          frame #2 {
            n127 = for {
              N: 7 -> [_]
              tunnel: [w1587] -> w1580
              tunnel: [w1588] -> _ mode=indexing
              tunnel: u8[] [68, 83, 67, 71, 50, 13, 10] ("unsigned byte array") -> [w1589] mode=indexing
              tunnel: [w1586] -> w1576
              tunnel: w1573 -> [w1585]
              w1587 = 1000 ("Timeout (ms)")
              n128 = xnode "FPGA I/O Method Node"("error in"=w1585, "Data"=w1589, "Timeout (ms)"=w1587) -> ("error out"=w1586:errorcluster, "Timed Out"=w1588:bool)  [unwired: 1 in, 1 out]
            }
            n129 = for {
              N: 12 -> [_]
              tunnel: w1580 -> [w1584]
              tunnel: [w1583] -> w1574 mode=indexing
              tunnel: w1576 -> [w1582]
              tunnel: [w1581] -> w1575
              n130 = xnode "FPGA I/O Method Node"("error in"=w1582, "Timeout (ms)"=w1584) -> ("error out"=w1581:errorcluster, "Data"=w1583:u8)  [unwired: 1 in, 2 out]
            }
            "R45 Vac Cluster 3 Convectron 2" <- w1574
          }
          frame #3 {
            n131 = for {
              N: 7 -> [_]
              tunnel: [w1604] -> w1597
              tunnel: [w1606] -> _ mode=indexing
              tunnel: u8[] [68, 83, 73, 71, 50, 13, 10] ("unsigned byte array") -> [w1605] mode=indexing
              tunnel: [w1603] -> w1592
              tunnel: w1590 -> [w1602]
              w1604 = 1000 ("Timeout (ms)")
              n132 = xnode "FPGA I/O Method Node"("error in"=w1602, "Data"=w1605, "Timeout (ms)"=w1604) -> ("error out"=w1603:errorcluster, "Timed Out"=w1606:bool)  [unwired: 1 in, 1 out]
            }
            n133 = for {
              N: 12 -> [_]
              tunnel: w1597 -> [w1601]
              tunnel: [w1600] -> w1593 mode=indexing
              tunnel: w1592 -> [w1599]
              tunnel: [w1598] -> w1591 mode=indexing
              n134 = xnode "FPGA I/O Method Node"("error in"=w1599, "Timeout (ms)"=w1601) -> ("error out"=w1598:errorcluster, "Data"=w1600:u8)  [unwired: 1 in, 2 out]
            }
            "R45 Vac Cluster 3 Ion Gauge 2" <- w1593
          }
        }
        n135 = Merge Errors(w1537, w1536, w1535, w1534) -> (w1533:errorcluster)
      }
    }
    "R45 Vacuum Gauge 3 error" <- w1529
  }
  n136 = while {
    tunnel: w1 -> [w1608]
    stop <- FALSE stop-if-true
    # "R45 Vacuum gauge set #4: GP-307 Vacuum gauge controller"
    n137 = flat-sequence {
      tunnel: w1608 -> [w1616]
      tunnel: [w1611] -> w1607
      frame #0 {
        n138 = call "Loop Timer8"("Count(mSec)"=u32 2000 ("Count(Ticks)")) -> ()  [unwired: 1 out]
      }
      frame #1 {
        n139 = stacked-sequence {
          tunnel: [_ _ w1653 _] -> w1613
          tunnel: [_ _ _ w1669] -> w1612
          tunnel: w1616 -> [w1619 w1636 w1651 w1668]
          tunnel: [w1617 _ _ _] -> w1615
          tunnel: [_ w1635 _ _] -> w1614
          frame #0 {
            n140 = for {
              N: 7 -> [_]
              tunnel: [w1633] -> w1620
              tunnel: [w1632] -> _ mode=indexing
              tunnel: u8[] [68, 83, 73, 71, 49, 13, 10] ("unsigned byte array") -> [w1631] mode=indexing
              tunnel: w1619 -> [w1630]
              tunnel: [w1629] -> w1618
              w1633 = 1000 ("Timeout (ms)")
              n141 = xnode "FPGA I/O Method Node"("error in"=w1630, "Data"=w1631, "Timeout (ms)"=w1633) -> ("error out"=w1629:errorcluster, "Timed Out"=w1632:bool)  [unwired: 1 in, 1 out]
            }
            n142 = for {
              N: 12 -> [_]
              tunnel: w1620 -> [w1628]
              tunnel: [w1627] -> w1621 mode=indexing
              tunnel: w1618 -> [w1626]
              tunnel: [w1625] -> w1617 mode=indexing
              n143 = xnode "FPGA I/O Method Node"("error in"=w1626, "Timeout (ms)"=w1628) -> ("error out"=w1625:errorcluster, "Data"=w1627:u8)  [unwired: 1 in, 2 out]
            }
            "R45 Vac Cluster 4 Ion Gauge 1" <- w1621
          }
          frame #1 {
            n144 = for {
              N: 7 -> [_]
              tunnel: [w1649] -> w1641
              tunnel: [w1648] -> _ mode=indexing
              tunnel: u8[] [68, 83, 67, 71, 49, 13, 10] ("unsigned byte array") -> [w1650] mode=indexing
              tunnel: w1636 -> [w1647]
              tunnel: [w1646] -> w1634
              w1649 = 1000 ("Timeout (ms)")
              n145 = xnode "FPGA I/O Method Node"("error in"=w1647, "Data"=w1650, "Timeout (ms)"=w1649) -> ("error out"=w1646:errorcluster, "Timed Out"=w1648:bool)  [unwired: 1 in, 1 out]
            }
            n146 = for {
              N: 12 -> [_]
              tunnel: w1641 -> [w1645]
              tunnel: [w1644] -> w1637 mode=indexing
              tunnel: w1634 -> [w1643]
              tunnel: [w1642] -> w1635 mode=indexing
              n147 = xnode "FPGA I/O Method Node"("error in"=w1643, "Timeout (ms)"=w1645) -> ("error out"=w1642:errorcluster, "Data"=w1644:u8)  [unwired: 1 in, 2 out]
            }
            "R45 Vac Cluster 4 Convectron 1" <- w1637
          }
          frame #2 {
            n148 = for {
              N: 7 -> [_]
              tunnel: [w1665] -> w1658
              tunnel: [w1666] -> _ mode=indexing
              tunnel: u8[] [68, 83, 67, 71, 50, 13, 10] ("unsigned byte array") -> [w1667] mode=indexing
              tunnel: [w1664] -> w1654
              tunnel: w1651 -> [w1663]
              w1665 = 1000 ("Timeout (ms)")
              n149 = xnode "FPGA I/O Method Node"("error in"=w1663, "Data"=w1667, "Timeout (ms)"=w1665) -> ("error out"=w1664:errorcluster, "Timed Out"=w1666:bool)  [unwired: 1 in, 1 out]
            }
            n150 = for {
              N: 12 -> [_]
              tunnel: w1658 -> [w1662]
              tunnel: [w1661] -> w1652 mode=indexing
              tunnel: w1654 -> [w1660]
              tunnel: [w1659] -> w1653
              n151 = xnode "FPGA I/O Method Node"("error in"=w1660, "Timeout (ms)"=w1662) -> ("error out"=w1659:errorcluster, "Data"=w1661:u8)  [unwired: 1 in, 2 out]
            }
            "R45 Vac Cluster 4 Convectron 2" <- w1652
          }
          frame #3 {
            n152 = for {
              N: 7 -> [_]
              tunnel: [w1682] -> w1675
              tunnel: [w1684] -> _ mode=indexing
              tunnel: u8[] [68, 83, 73, 71, 50, 13, 10] ("unsigned byte array") -> [w1683] mode=indexing
              tunnel: [w1681] -> w1670
              tunnel: w1668 -> [w1680]
              w1682 = 1000 ("Timeout (ms)")
              n153 = xnode "FPGA I/O Method Node"("error in"=w1680, "Data"=w1683, "Timeout (ms)"=w1682) -> ("error out"=w1681:errorcluster, "Timed Out"=w1684:bool)  [unwired: 1 in, 1 out]
            }
            n154 = for {
              N: 12 -> [_]
              tunnel: w1675 -> [w1679]
              tunnel: [w1678] -> w1671 mode=indexing
              tunnel: w1670 -> [w1677]
              tunnel: [w1676] -> w1669 mode=indexing
              n155 = xnode "FPGA I/O Method Node"("error in"=w1677, "Timeout (ms)"=w1679) -> ("error out"=w1676:errorcluster, "Data"=w1678:u8)  [unwired: 1 in, 2 out]
            }
            "R45 Vac Cluster 4 Ion Gauge 2" <- w1671
          }
        }
        n156 = Merge Errors(w1615, w1614, w1613, w1612) -> (w1611:errorcluster)
      }
    }
    "R45 Vacuum Gauge 4 error" <- w1607
  }
